vi "Write IndexQ.vi"(8 "error in (no error)":errorcluster, 10 "IndexQ":refnum<queue>, 11 "CO2 Actor in":refnum<class "CO2 Actor.lvclass">) -> (0 "error out":errorcluster, 3 "CO2 Actor out":refnum<class "CO2 Actor.lvclass">)   [LabVIEW 2015, in "cRIO-Carbondioxide.lvlib" / "CO2-Actor.lvlib" / "CO2 Actor.lvclass"]
uses:
  CO2 Actor.lvclass
  CO2 Actor.lvclass/CO2 Actor.ctl
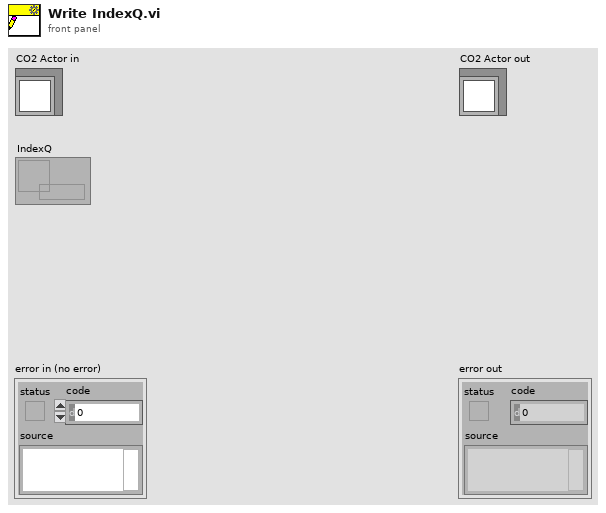
[diagram p1: front panel]
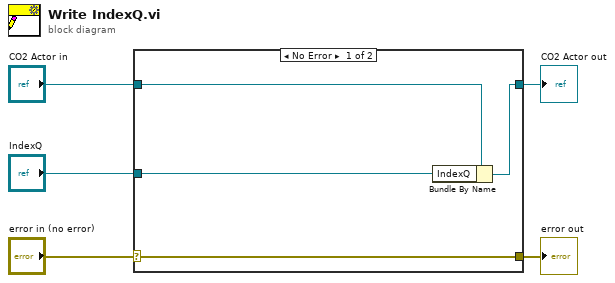
[diagram p0: block diagram]
diagram:
  n1 = case shown="No Error" "error in (no error)" {
    selector: "error in (no error)" -> [w9 w10]
    tunnel: [w9 w10] -> w4
    tunnel: [w7 w11] -> w2
    tunnel: "CO2 Actor in" -> [w8 w11]
    tunnel: "IndexQ" -> [w6 _]
    frame No Error {
      n2 = Bundle By Name(cluster=w8, "IndexQ"=w6) -> (w7:refnum<class "CO2 Actor.lvclass">)
    }
    frame Error {
    }
  }
  "error out" <- w4
  "CO2 Actor out" <- w2
